vi "set_element_at.vi"(6 "id chain":string[](array[string]), 8 "error in (no error)":errorcluster, 9 "element":refnum<class "XMLElement.lvclass">, 10 "key chain":string[](array[string]), 11 "Element in":refnum<class "XMLElement.lvclass">) -> (0 "error out":errorcluster, 3 "Element out":refnum<class "XMLElement.lvclass">)   [LabVIEW 2010, in "XMLElement.lvclass"]
uses:
  XMLElement.lvclass
  XMLElement.lvclass/XMLElement.ctl
  Program Files/National Instruments/LabVIEW 2010/resource/objmgr/DOMUserDefRef.rc
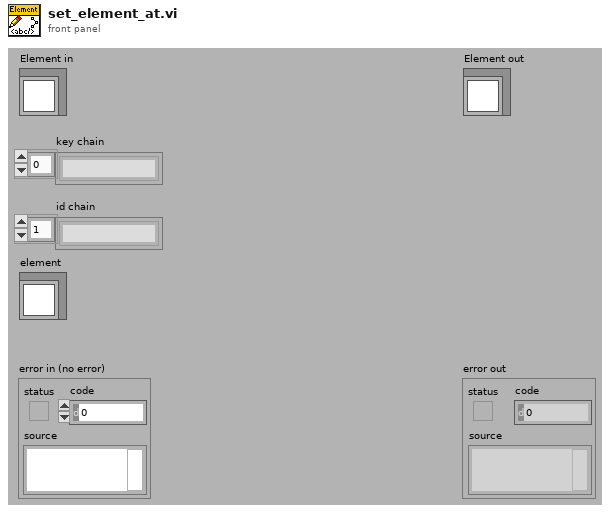
[diagram p1: front panel]
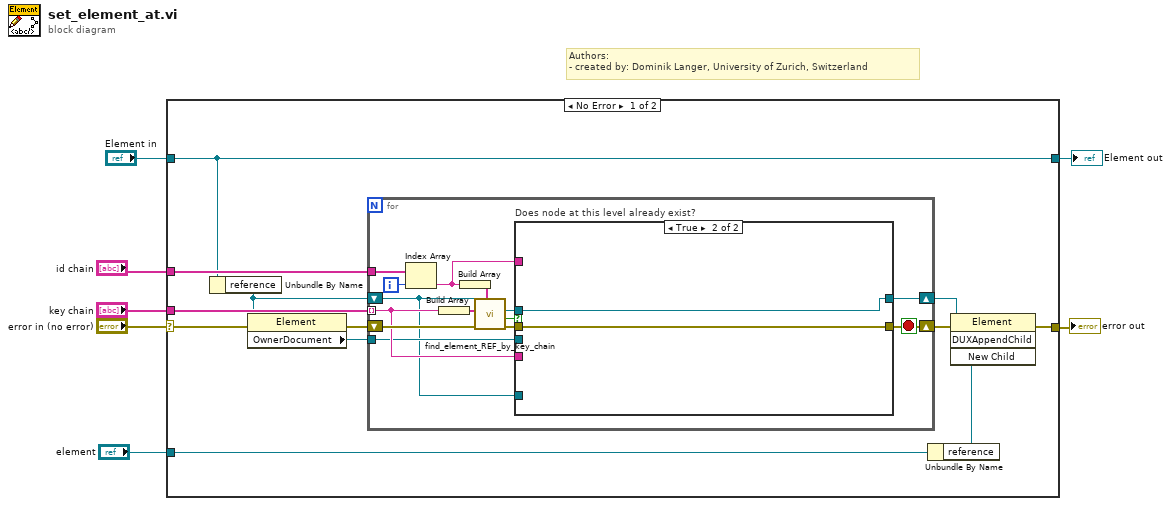
[diagram p0: block diagram]
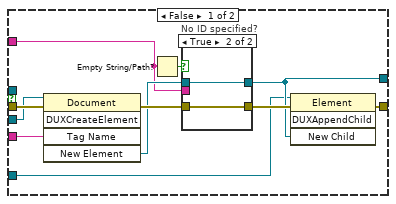
[diagram p2: hidden frame]
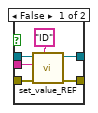
[diagram p3: hidden frame]
diagram:
  # "Authors: \n- created by: Dominik Langer, University of Zurich, Switzerland"
  n1 = case shown="No Error" "error in (no error)" {
    selector: "error in (no error)" -> [w11 w55]
    tunnel: [w16 w55] -> w6
    tunnel: [w14 w54] -> w4
    tunnel: "Element in" -> [w14 w54]
    tunnel: "key chain" -> [w15 _]
    tunnel: "id chain" -> [w18 _]
    tunnel: "element" -> [w17 _]
    frame No Error {
      n2 = Unbundle By Name(w14) -> ("reference"=w9:refnum<k20>)
      n3 = property class="Element"(reference=w9, error in=w11) -> (error out=w10:errorcluster, "OwnerDocument"=w8:refnum<k20>)  [unwired: 1 out]
      n4 = for {
        shift-right: [w22] -> _
        shift-left: w10 -> [w30]
        tunnel: w15 -> [w26] mode=indexing
        tunnel: w18 -> [w25]
        shift-right: [w32] -> w12
        shift-left: w9 -> [w20]
        tunnel: w8 -> [w21]
        i -> [w23]
        stop <- w22 stop-if-true
        n5 = Index Array(array=w25, index=w23) -> (element=w24:string)
        n6 = Build Array(w26) -> (w31:string[])
        n7 = Build Array(w24) -> (w28:string[])
        n8 = call "find_element_REF_by_key_chain.vi"("id chain"=w28, "error in (no error)"=w30, "key chain"=w31, "element ref"=w20) -> ("error out"=w29:errorcluster, "found?"=w27:bool, "subelement ref"=w19:refnum<k20>)  [unwired: 5 in]
        n9 = case "Does node at this level already exist?" shown="True" w27 {
          tunnel: w29 -> [w41 w53]
          tunnel: [w36 w52] -> w32
          tunnel: [w43 w53] -> w22
          tunnel: w26 -> [w42 _]
          tunnel: w24 -> [w35 _]
          tunnel: w21 -> [w40 _]
          tunnel: w20 -> [w33 _]
          tunnel: w19 -> [_ w52]
          frame False {
            n10 = invoke class="Document" method="DUXCreateElement"(reference=w40, error in=w41, "Tag Name"=w42) -> (error out=w39:errorcluster, "New Element"=w37:refnum<k20>)  [unwired: 2 in, 3 out]
            n11 = Empty String/Path?(string/path=w35) -> (empty?=w34:bool)
            n12 = case "No ID specified?" shown="True" w34 {
              tunnel: w37 -> [w46 w50]
              tunnel: w39 -> [w49 w51]
              tunnel: [w48 w51] -> w38
              tunnel: w35 -> [w44 _]
              tunnel: [w47 w50] -> w36
              frame False {
                n13 = call "set_value_REF.vi"("attribute name"="ID" ("Name"), "error in (no error)"=w49, "value"=w44, "Element ref in"=w46) -> ("error out"=w48:errorcluster, "Element ref out"=w47:refnum<k20>)  [unwired: 6 in]
              }
              frame True {
              }
            }
            n14 = invoke class="Element" method="DUXAppendChild"(reference=w33, error in=w38, "New Child"=w36) -> (error out=w43:errorcluster)  [unwired: 1 in, 3 out]
          }
          frame True {
          }
        }
      }
      n15 = Unbundle By Name(w17) -> ("reference"=w13:refnum<k20>)
      n16 = invoke class="Element" method="DUXAppendChild"(reference=w12, error in=w10, "New Child"=w13) -> (error out=w16:errorcluster)  [unwired: 1 in, 3 out]
    }
    frame Error {
    }
  }
  "error out" <- w6
  "Element out" <- w4
